vi "Configure.vi"(8 "error in (no error)":errorcluster, 11 "1553 Component in":refnum<class "1553 Component.lvclass">) -> (0 "error out":errorcluster, 3 "1553 Component out":refnum<class "1553 Component.lvclass">)   [LabVIEW 2020, in "BCI-1553 API.lvlib" / "1553 Component.lvclass"]
doc: "Parses the component configuration and pushes it to the component hardware."
uses:
  1553 Component.lvclass
  1553 Component.lvclass/1553 Component.ctl
  1553 SubComponent/1553 SubComponent.lvclass
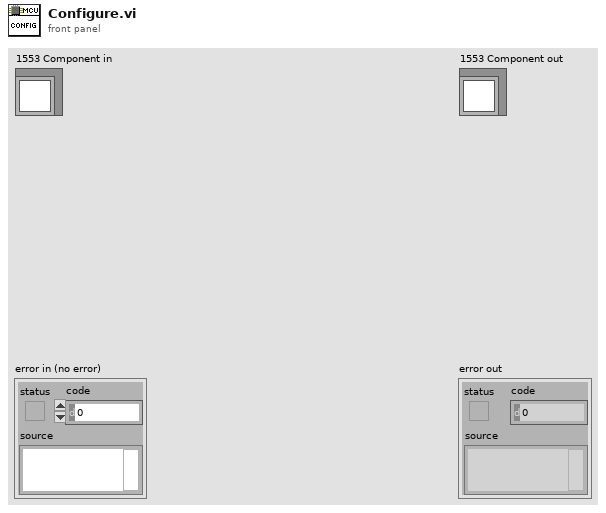
[diagram p1: front panel]
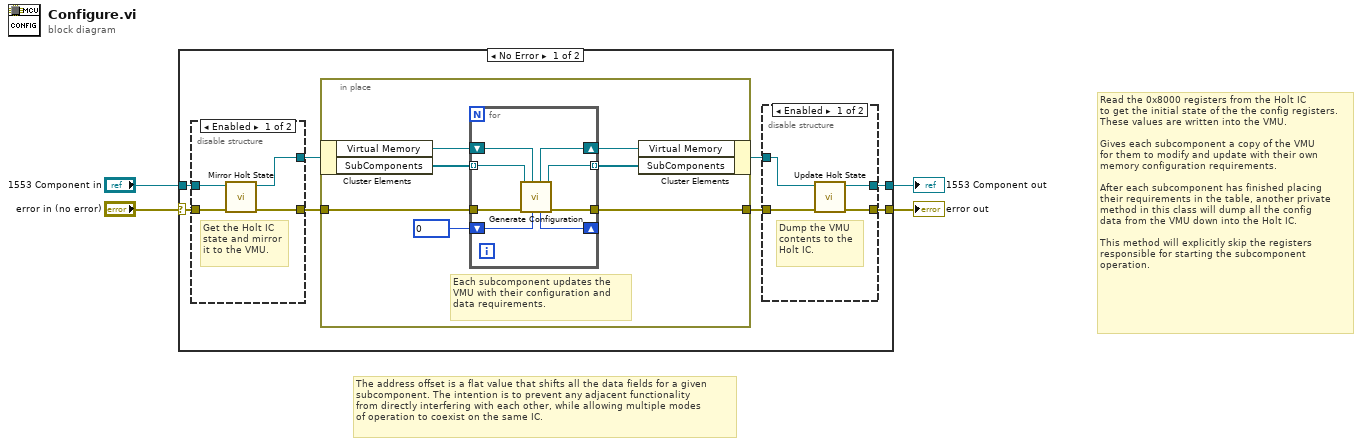
[diagram p0: block diagram]
diagram:
  # "The address offset is a flat value that shifts all the data fields for a given\nsubcomponent. The intention is to prevent any adjacent functionality \nfrom directly interfering with each other, while allowing multiple modes\nof operation to coexist on the same IC."
  # "Read the 0x8000 registers from the Holt IC\nto get the initial state of the the config registers.\nThese values are written into the VMU.\n\nGives each subcomponent a copy of the VMU\nfor them to modify and update with their own\nmemory configuration requirements.\n\nAfter each subcomponent has finished placing\ntheir requirements in the table, another private\nmethod in this class will dump all the config\ndata from the VMU down into the Holt IC.\n\nThis method will explicitly skip the registers\nresponsible for starting the subcomponent\noperation."
  n1 = case shown="No Error" "error in (no error)" {
    selector: "error in (no error)" -> [w12 w41]
    tunnel: [w6 w41] -> w3
    tunnel: [w7 w40] -> w1
    tunnel: "1553 Component in" -> [w11 w40]
    frame No Error {
      n2 = disable-structure shown="Enabled" {
        disable-tunnel: w12 -> [w22 w23]
        disable-tunnel: w11 -> [w21 w24]
        disable-tunnel: [w20 w23] -> w10
        disable-tunnel: [w19 w24] -> w9
        frame Enabled {
          # "Get the Holt IC \nstate and mirror\nit to the VMU."
          n3 = call "Mirror Holt State.vi"("error in (no error)"=w22, "1553 Component in"=w21) -> ("error out"=w20:errorcluster, "1553 Component out"=w19:refnum<class "1553 Component.lvclass">)  [unwired: 8 in]
        }
        frame Disabled {
        }
      }
      n4 = in-place {
        in-place-border: w10 -> [w31]
        in-place-border: [w28] -> w5
        # "Each subcomponent updates the\nVMU with their configuration and\ndata requirements."
        n5 = in-place-cluster #1(w9) -> ("Virtual Memory"=w29:refnum<class "Virtual Memory Unit.lvclass">, "SubComponents"=w30:refnum<class "1553 SubComponent.lvclass">[])
        n6 = for {
          tunnel: w31 -> [w36]
          tunnel: w30 -> [w39] mode=indexing
          shift-right: [w37] -> w26
          shift-left: w29 -> [w38]
          tunnel: [w35] -> w28
          tunnel: [w34] -> w27 mode=indexing
          shift-right: [w33] -> _
          shift-left: u16 0 ("Starting Address Offset") -> [w32]
          n7 = call-dynamic "Generate Configuration.vi"("Starting Address Offset"=w32, "Virtual Memory Unit in"=w38, "error in (no error)"=w36, "1553 SubComponent in"=w39) -> ("error out"=w35:errorcluster, "1553 SubComponent out"=w34:refnum<class "1553 SubComponent.lvclass">, "Next Address Offset"=w33:u16, "Virtual Memory Unit out"=w37:refnum<class "Virtual Memory Unit.lvclass">)  [unwired: 3 in, 1 out]
        }
        n8 = in-place-cluster #1("Virtual Memory"=w26, "SubComponents"=w27) -> (w8:refnum<class "1553 Component.lvclass">)
      }
      n9 = disable-structure shown="Enabled" {
        disable-tunnel: w8 -> [w16 w18]
        disable-tunnel: [w15 w18] -> w7
        disable-tunnel: [w14 w17] -> w6
        disable-tunnel: w5 -> [w13 w17]
        frame Enabled {
          # "Dump the VMU\ncontents to the \nHolt IC."
          n10 = call "Update Holt State.vi"("error in (no error)"=w13, "1553 Component in"=w16) -> ("error out"=w14:errorcluster, "1553 Component out"=w15:refnum<class "1553 Component.lvclass">)  [unwired: 8 in]
        }
        frame Disabled {
        }
      }
    }
    frame Error {
    }
  }
  "error out" <- w3
  "1553 Component out" <- w1
